vi "testCAN 2.vi"() -> ()   [LabVIEW 2015]
uses:
  <vilib>/Utility/Variable/NI_VariableUtilities.lvlib
  <vilib>/Utility/inputDevices.llb/joystickAcquire.vi
  CANFrameControl.ctl
panel:
  out "ramki can":string
  in  "stop 5":bool
  out "data string":string
  out "# pending insert":i32
  out "# pending remove":i32
  out "# elements in queue":i32
  out "appended array":string[](array[string])
  in  "stop 4":bool
  out "ilosc mesag":dbl
  in  "stop 3":bool
  in  "Boolean":bool
  out "Numeric 2":i32
  in  "stop event":bool
  in  "Tab Control":T1(tab)
  in  "Przód":T2
  out "size(s)":i32[](array[numeric])
  in  "identifier 2":u32 format="%x"
  in  "identifier":u32 format="%x"
  out "output 5":u16
  out "output 4":u16
  out "element 2":string
  out "element":string
  out "output 2":u16
  out "output 3":u16
  in  "device index":i32
  in  "Number of Frames to Display":i32=15
  out "Frames":string[][](table)
  in  "stop":bool
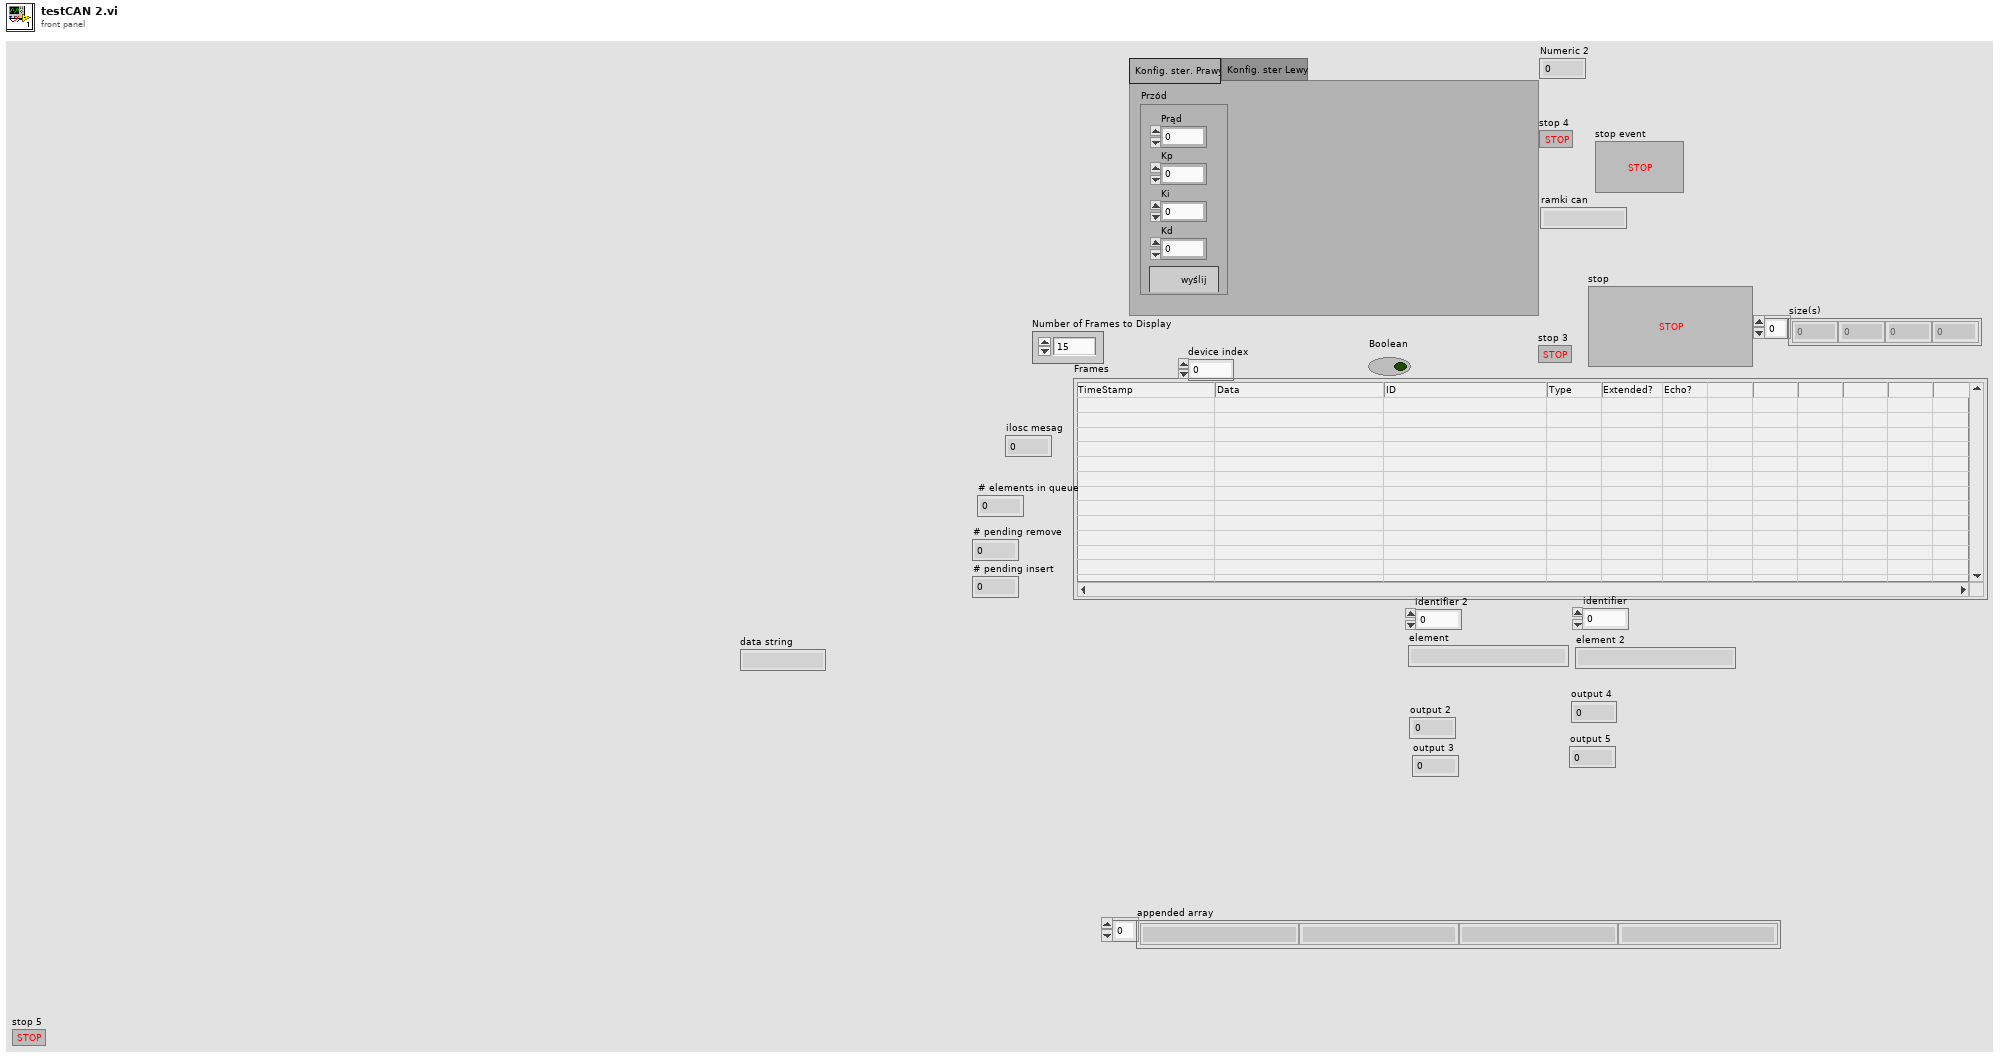
[diagram p1: front panel]
types:
  T1 = enum32{"Konfig. ster. Prawy", "Konfig. ster Lewy"}
  T2 = cluster{"Prąd":u16, "Kp":u16, "Ki":u16, "Kd":u16, "OK Button":bool}
  T3 = typedef "CANFrameControl.ctl" = cluster{"identifier":u32, "extended?":bool, "type":u8, "payload":u8[]}
  T4 = cluster{"X axis":i32, "Y axis":i32, "Z axis":i32, "X axis rotation":i32, "Y axis rotation":i32, "Z axis rotation":i32, "U axis":i32, "V axis":i32}
  T5 = cluster{"button 1":bool, "button 2":bool, "button 3":bool, "button 4":bool, "button 5":bool, "button 6":bool, "button 7":bool, "button 8":bool, "button 9":bool, "button 10":bool, "button 11":bool, "button 12":bool, "button 13":bool, "button 14":bool, "button 15":bool, "button 16":bool, "button 17":bool, "button 18":bool, "button 19":bool, "button 20":bool, "button 21":bool, "button 22":bool, "button 23":bool, "button 24":bool, "button 25":bool, "button 26":bool, "button 27":bool, "button 28":bool, "button 29":bool, "button 30":bool, "button 31":bool, "button 32":bool}
  T6 = typedef "wyj auto.ctl" = cluster{"AUTO ?":bool, "zadany czas":bool, "Time has Elapsed":bool, "Elapsed Time (s)":dbl, "seconds since 1Jan1904":timestamp}
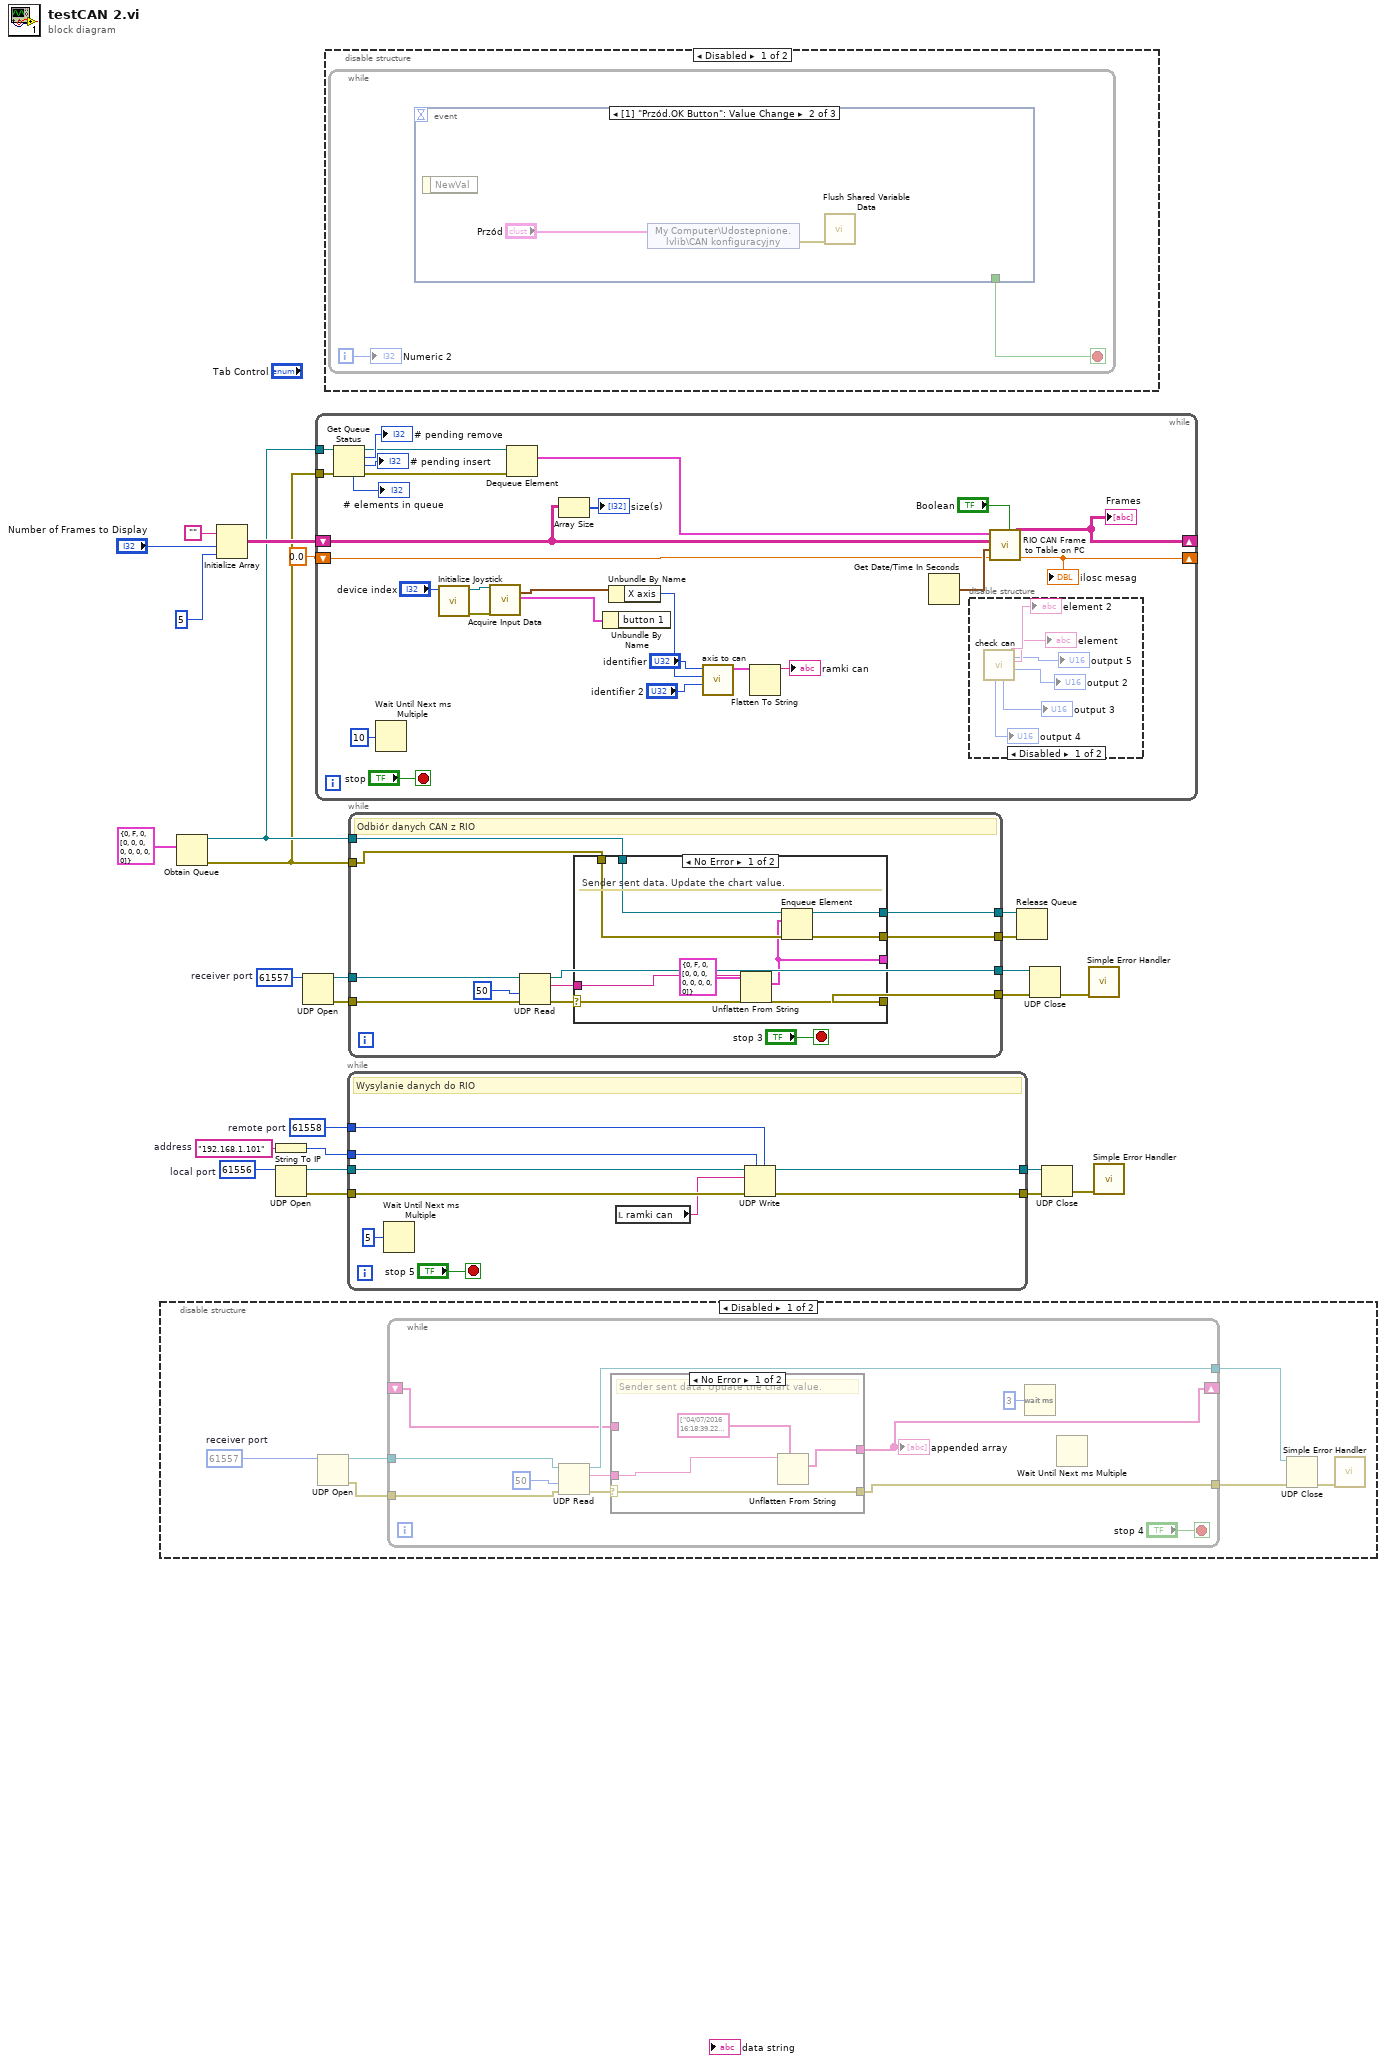
[diagram p0: block diagram]
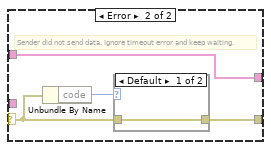
[diagram p2: hidden frame]
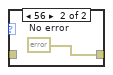
[diagram p3: hidden frame]
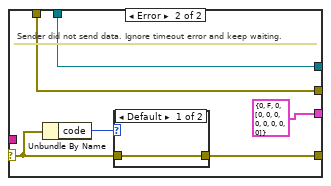
[diagram p5: hidden frame]
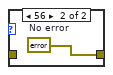
[diagram p6: hidden frame]
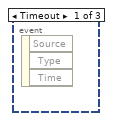
[diagram p7: hidden frame]
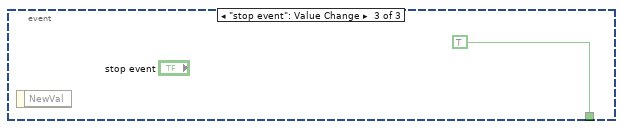
[diagram p8: hidden frame]
diagram:
  w1 = u16 61558  # remote port
  w9 = u16 61556  # local port
  w8 = "192.168.1.101"  # address
  w20 = u16 61557  # receiver port
  n1 = disable-structure shown="Disabled" {
    frame Disabled {
      w26 = u16 61557  # receiver port
      n2 = UDP Open(11:w26) -> (port=w28:refnum<k16>, 0:w29:errorcluster)  [unwired: 4 in, 1 out]
      n3 = while {
        tunnel: w28 -> [w39]
        tunnel: w29 -> [w38]
        tunnel: [w37] -> w30
        tunnel: [w34] -> w31
        shift-right: [w33] -> _
        shift-left: _ -> [w32]
        stop <- "stop 4" stop-if-true
        n4 = UDP Read(connection ID=w39, timeout ms (25000)=50, 8:w38) -> (data out=w41:string, error out=w40:errorcluster, 3:w34:refnum<k16>)  [unwired: 3 out]
        n5 = case shown="No Error" w40 {
          selector: w40 -> [w46 w49]
          tunnel: w41 -> [w45 _]
          tunnel: [w46 w48] -> w37
          tunnel: [w44 w47] -> w33
          tunnel: w32 -> [_ w47]
          frame No Error {
            # "Sender sent data. Update the chart value."
            n6 = Unflatten From String(type=string[] ["04/07/2016 16:18:39.223313", " 17\t 17\t 17\t 17\t 17\t 17\t 17\t 17\n", "1", "CAN Data", "No"] ("appended array"), binary string=w45) -> (value=w44:string[])  [unwired: 3 in, 2 out]
          }
          frame Error {
            # "Sender did not send data. Ignore timeout error and keep waiting."
            n7 = Unbundle By Name(w49) -> ("code"=w50:i32)
            n8 = case shown="Default" w50 {
              tunnel: w49 -> [w51 _]
              tunnel: [w51 w52] -> w48
              frame Default {
              }
              frame 56 {
                w52 = errorcluster {"status"=FALSE, "code"=0, "source"=""}  # No error
              }
            }
          }
        }
        "appended array" <- w33
        n9 = Wait (ms)(milliseconds to wait=u32 3 ("millisecond multiple")) -> ()  [unwired: 1 out]
        n10 = Wait Until Next ms Multiple() -> ()  [unwired: 1 in, 1 out]
      }
      n11 = UDP Close(connection ID=w31, 8:w30) -> (error out=w27:errorcluster)  [unwired: 1 out]
      n12 = call <vilib>:"Simple Error Handler.vi"("error in (no error)"=w27) -> ()  [unwired: 1 in, 8 out]
    }
    frame Enabled {
    }
  }
  n13 = Obtain Queue(element data type=T3 {"identifier"=0, "extended?"=FALSE, "type"=0, "payload"=[0, 0, 0, 0, 0, 0, 0, 0]} ("CAN frame")) -> (queue out=w11:refnum<queue>, error out=w10:errorcluster)  [unwired: 4 in, 1 out]
  n14 = Initialize Array("" ("Empty String Constant"), "Number of Frames to Display", 5 ("dimension size")) -> (w22:string[][])
  n15 = String To IP(1:w8) -> (0:w2:u32)
  n16 = UDP Open(11:w9) -> (port=w6:refnum<k16>, 0:w5:errorcluster)  [unwired: 4 in, 1 out]
  n17 = UDP Open(11:w20) -> (port=w18:refnum<k16>, 0:w17:errorcluster)  [unwired: 4 in, 1 out]
  n18 = while {
    shift-right: [w66] -> _
    shift-left: w22 -> [w68]
    shift-right: [w65] -> _
    shift-left: 0.0 ("Numeric") -> [w64]
    tunnel: w11 -> [w60]
    tunnel: w10 -> [w59]
    stop <- "stop" stop-if-true
    n19 = Get Queue Status(queue=w60, error in (no error)=w59) -> (queue out=w55:refnum<queue>, # pending remove=→"# pending remove":i32, # pending insert=→"# pending insert":i32, error out=w61:errorcluster, # elements in queue=→"# elements in queue":i32)  [unwired: 1 in, 3 out]
    n20 = Wait Until Next ms Multiple(millisecond multiple=u32 10 ("milliseconds to wait")) -> ()  [unwired: 1 out]
    n21 = call <vilib>:"Initialize Joystick.vi"("device index"="device index") -> ("error out"=w77:errorcluster, "device ID"=w78:refnum<k1>)  [unwired: 9 in]
    n22 = call-poly <vilib>:"Acquire Input Data.vi"("device ID"=w78, "error in (no error)"=w77) -> ("axis info"=w75:T4, "button info"=w74:T5)  [unwired: 13 in, 3 out]
    n23 = Dequeue Element(queue=w55, error in (no error)=w61) -> (element=w62:T3)  [unwired: 1 in, 3 out]
    n24 = Array Size(array=w68) -> (size(s)=→"size(s)":i32[])
    n25 = Unbundle By Name(w74) -> ()  [unwired: 1 out]
    n26 = Unbundle By Name(w75) -> ("X axis"=w73:i32)
    n27 = call "axis to can.vi"("wej  ID"="identifier 2", "wej wagi"=w73, "ROS in"="identifier") -> ("wyj auto"=w54:T6)  [unwired: 5 in, 3 out]
    n28 = Flatten To String(anything=w54) -> (data string=→"ramki can":string)  [unwired: 3 in, 2 out]
    n29 = Get Date/Time In Seconds() -> (seconds since 1Jan1904=w69:timestamp)
    n30 = disable-structure shown="Disabled" {
      frame Disabled {
        n31 = call "check can.vi"() -> ("Numeric"=→"output 2":u16, "element"=→"element":string, "element 2"=→"element 2":string, "output 3"=→"output 3":u16, "output 5"=→"output 5":u16, "output 4"=→"output 4":u16)  [unwired: 6 in]
      }
      frame Enabled {
      }
    }
    n32 = call "RIO CAN Frame to Table on PC.vi"("Boolean"="Boolean", "x"=w64, "timestamp"=w69, "Input Array"=w68, "CAN frame"=w62) -> ("Numeric"=w65:dbl, "Output Array"=w66:string[][])  [unwired: 2 in, 3 out]
    "Frames" <- w66
    "ilosc mesag" <- w65
  }
  n33 = disable-structure shown="Disabled" {
    frame Disabled {
      n34 = while {
        i -> [w86]
        stop <- w87 stop-if-true
        n35 = event shown="[1] \"Przód.OK Button\": Value Change" {
          selector: _ -> [_ _ _]
          dyn-events: _ -> [_ _ _]
          timeout: _ -> [_ _ _]
          tunnel: [_ _ TRUE] -> w87
          event Timeout {
            n36 = event-data() -> ()  [unwired: 1 in, 3 out]
          }
          event "Przód.OK Button": Value Change {
            n37 = event-data() -> ()  [unwired: 1 in, 1 out]
            n38 = shared-variable "My Computer\\Udostepnione.lvlib\\CAN konfiguracyjny"("Przód") -> (error out=w88:errorcluster)  [unwired: 1 in]
            n39 = call <vilib>:"Flush Shared Variable Data.vi"("error in (no error)"=w88) -> ()  [unwired: 10 in, 1 out]
          }
          event "stop event": Value Change {
            n40 = event-data() -> ()  [unwired: 1 in, 1 out]
          }
        }
        "Numeric 2" <- w86
      }
    }
    frame Enabled {
    }
  }
  n41 = while {
    tunnel: w6 -> [w99]
    tunnel: w5 -> [w98]
    tunnel: [w96] -> w4
    tunnel: [w95] -> w3
    tunnel: w2 -> [w94]
    tunnel: w1 -> [w93]
    stop <- "stop 5" stop-if-true
    # "Wysylanie danych do RIO"
    n42 = Wait Until Next ms Multiple(millisecond multiple=u32 5) -> ()  [unwired: 1 out]
    n43 = local read "ramki can"() -> (w91:string)
    n44 = UDP Write(address=w94, port or service name=w93, connection ID=w99, data in=w91, 8:w98) -> (error out=w95:errorcluster, 3:w96:refnum<k16>)  [unwired: 1 in]
  }
  n45 = while {
    tunnel: w18 -> [w108]
    tunnel: w17 -> [w107]
    tunnel: [w106] -> w16
    tunnel: [w104] -> w15
    tunnel: [w102] -> w14
    tunnel: [w100] -> w13
    tunnel: w11 -> [w103]
    tunnel: w10 -> [w101]
    stop <- "stop 3" stop-if-true
    # "Odbiór danych CAN z RIO"
    n46 = UDP Read(connection ID=w108, timeout ms (25000)=50, 8:w107) -> (data out=w110:string, error out=w109:errorcluster, 3:w104:refnum<k16>)  [unwired: 3 out]
    n47 = case shown="No Error" w109 {
      selector: w109 -> [w119 w124]
      tunnel: w110 -> [w118 _]
      tunnel: [w119 w123] -> w106
      tunnel: [w112 T3 {"identifier"=0, "extended?"=FALSE, "type"=0, "payload"=[0, 0, 0, 0, 0, 0, 0, 0]} ("CAN frame")] -> _
      tunnel: w103 -> [w116 w121]
      tunnel: [w115 w121] -> w102
      tunnel: w101 -> [w114 w120]
      tunnel: [w113 w120] -> w100
      frame No Error {
        # "Sender sent data. Update the chart value."
        n48 = Unflatten From String(type=T3 {"identifier"=0, "extended?"=FALSE, "type"=0, "payload"=[0, 0, 0, 0, 0, 0, 0, 0]} ("CAN frame"), binary string=w118) -> (value=w112:T3)  [unwired: 3 in, 2 out]
        n49 = Enqueue Element(queue=w116, element=w112, error in (no error)=w114) -> (queue out=w115:refnum<queue>, error out=w113:errorcluster)  [unwired: 1 in, 1 out]
      }
      frame Error {
        # "Sender did not send data. Ignore timeout error and keep waiting."
        n50 = Unbundle By Name(w124) -> ("code"=w125:i32)
        n51 = case shown="Default" w125 {
          tunnel: w124 -> [w126 _]
          tunnel: [w126 w127] -> w123
          frame Default {
          }
          frame 56 {
            w127 = errorcluster {"status"=FALSE, "code"=0, "source"=""}  # No error
          }
        }
      }
    }
  }
  n52 = Release Queue(queue=w14, error in (no error)=w13) -> ()  [unwired: 1 in, 3 out]
  n53 = UDP Close(connection ID=w15, 8:w16) -> (error out=w19:errorcluster)  [unwired: 1 out]
  n54 = UDP Close(connection ID=w4, 8:w3) -> (error out=w7:errorcluster)  [unwired: 1 out]
  n55 = call <vilib>:"Simple Error Handler.vi"("error in (no error)"=w19) -> ()  [unwired: 1 in, 8 out]
  n56 = call <vilib>:"Simple Error Handler.vi"("error in (no error)"=w7) -> ()  [unwired: 4 in, 5 out]
